vi "Joystick and Camera.vi"() -> ()   [LabVIEW 2016]
uses:
  Classes/Controller/Camera/Machine Vision.ctl
  Classes/Controller/I-O/I-O.lvclass
  Classes/Controller/Motion/Motion.lvclass
  Classes/Controller/Camera/Camera.lvclass
  Classes/Controller/Controller.lvclass
panel:
  out "x .and. y?":bool
  out "Array":dbl[](array[numeric])
  out "array w/ subset deleted":dbl[](array[numeric])
  in  "Go 3":bool
  in  "light":dbl=5.0
  in  "Change light":bool
  out "XYZTheta Out":dbl[](array[numeric])
  in  "Machine Vision":T1
  in  "Move 10cm Right":bool
  in  "Move 10cm Backward":bool
  in  "Move 10cm Forward":bool
  in  "Move 10cm Left":bool
  in  "Record Measurement":bool=TRUE
  in  "Dismount Silicon Tray":bool
  in  "Secure Silicon Tray":bool
  in  "Z Go":bool
  in  "Position":dbl
  in  "XYZTheta":dbl[](array[numeric])
  in  "Go":bool
  in  "Joystick":bool
  out "Sum":dbl[](array[numeric])
  out "Gantry":dbl[](array[numeric])
  in  "Stop":bool
  out "Image":T2(plugin-control)
  out "Camera":dbl[](array[numeric])
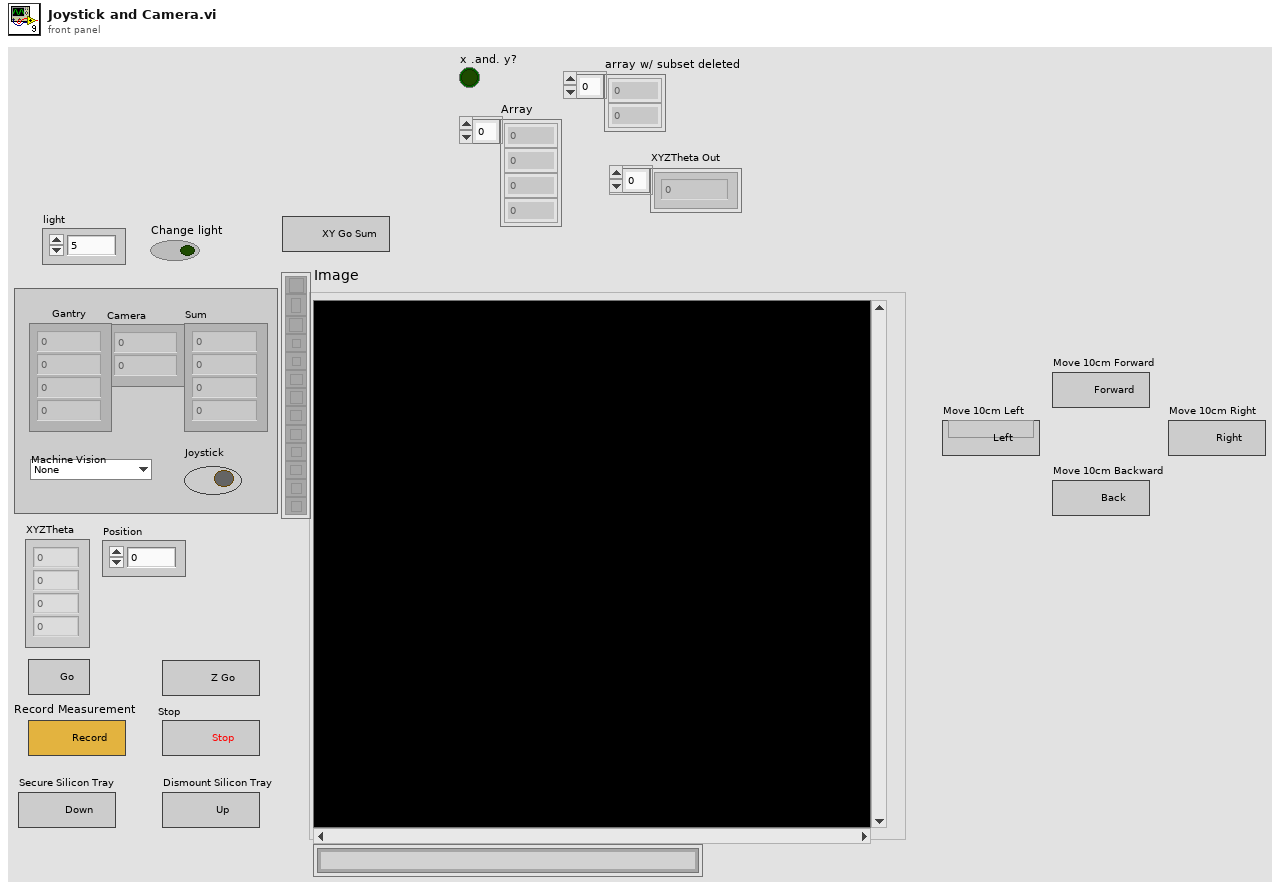
[diagram p1: front panel]
types:
  T1 = typedef "Camera.lvclass/Machine Vision.ctl" = enum16{"None", "Circle", "Tray Fiducials", "Tray Fiducials, top right", "HPK Silicon", "Hexaboard", "Corner (TL, BR)", "Corner (BL, TR)"}
  T2 = typedef "IMAQ Image.ctl" = refnum<image>
  T3 = typedef "Controller.lvclass/Controllers.ctl" = cluster{"I-O.lvclass":refnum<class "I-O.lvclass">, "Motion.lvclass":refnum<class "Motion.lvclass">, "Dispenser.lvclass":refnum<class "Dispenser.lvclass">}
  T4 = typedef "I-O.lvclass/Pin Map.ctl" = cluster{"Region Valves":i32[], "Extra Valves":dbl[][][], "Tool Primary Valve":i32, "Tool Secondary Valve":i32, "Region Sensors":i32[], "Extra Sensors":dbl[][][], "Tool Primary Sensor":dbl, "Tool Secondary Sensor":dbl, "Compression Sensor":dbl, "5V":i32}
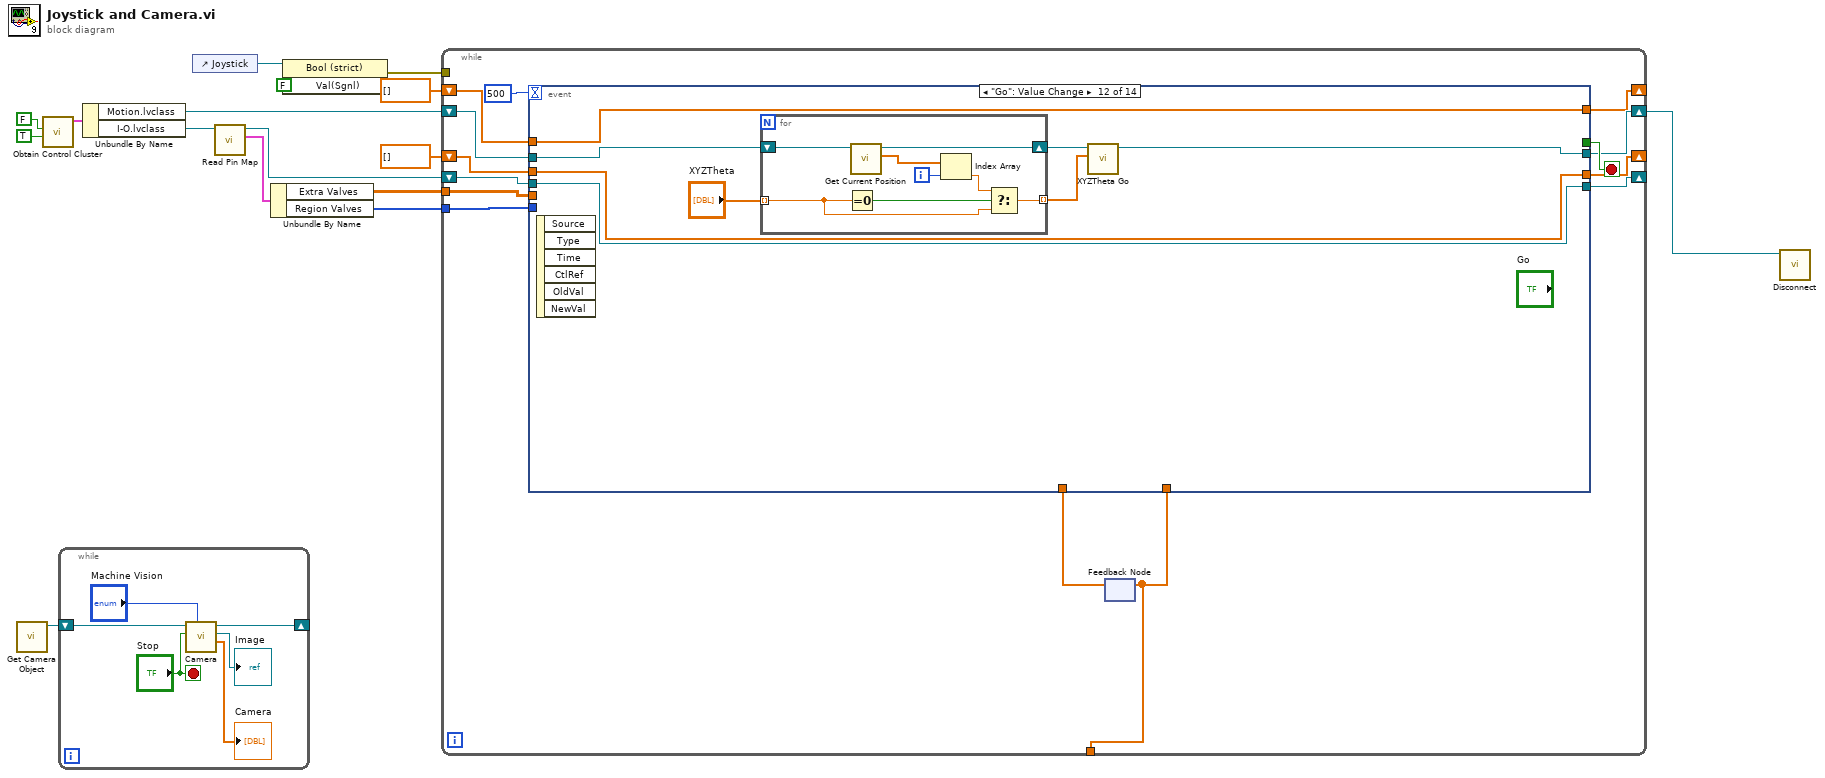
[diagram p0: block diagram]
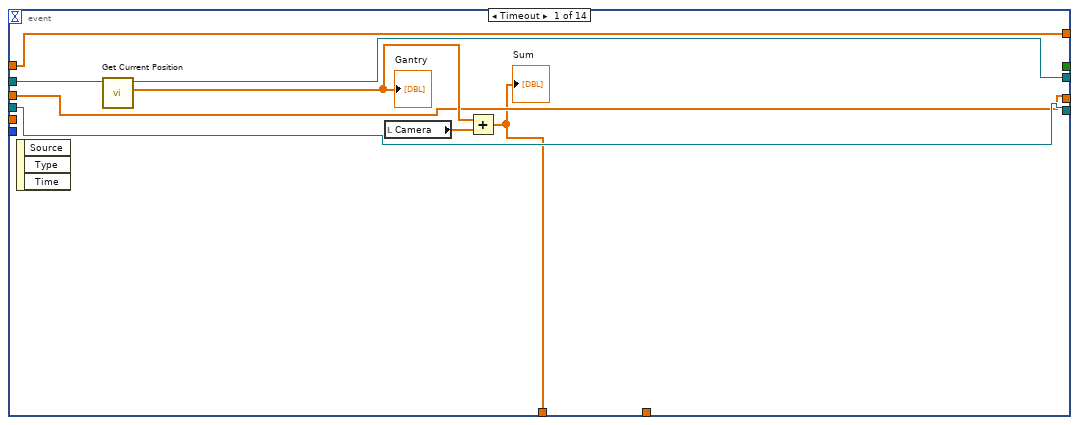
[diagram p2: hidden frame]
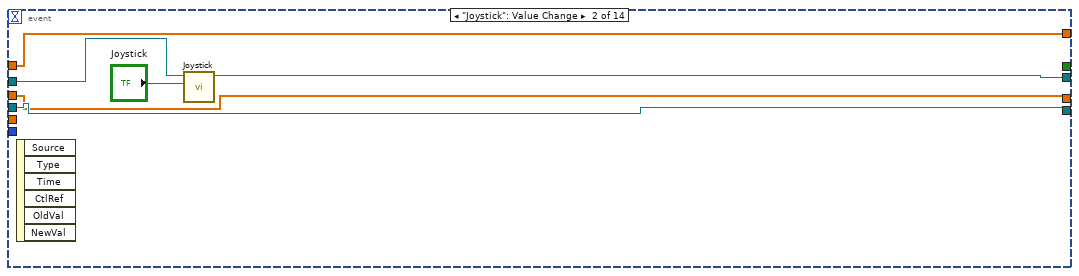
[diagram p3: hidden frame]
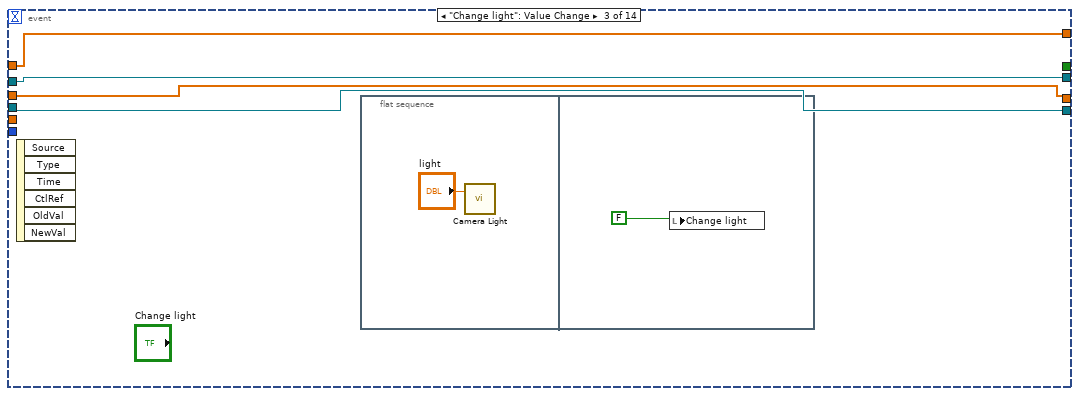
[diagram p4: hidden frame]
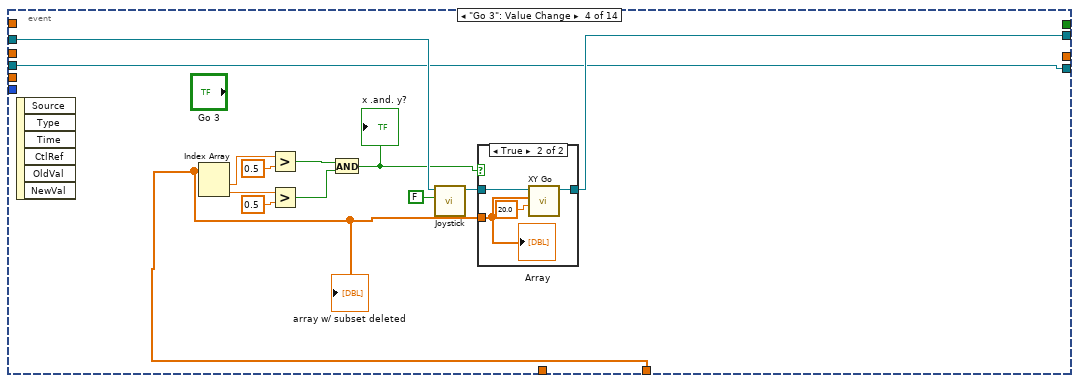
[diagram p5: hidden frame]
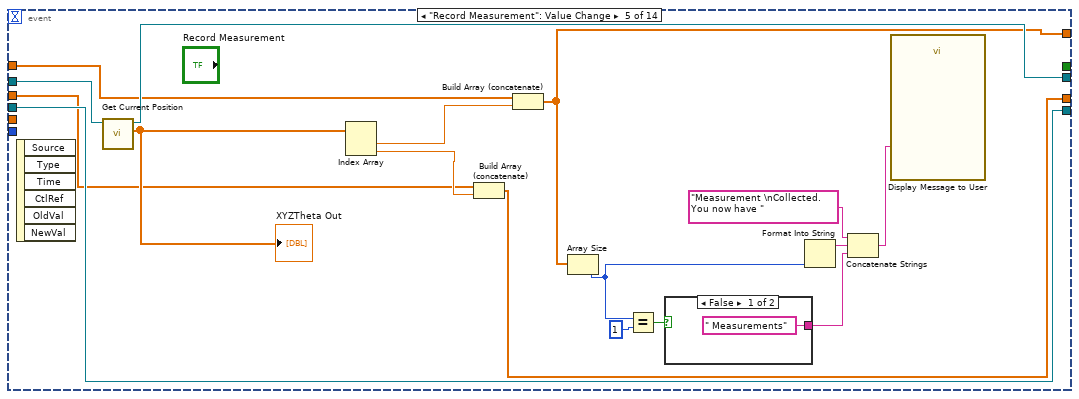
[diagram p7: hidden frame]
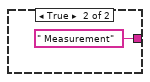
[diagram p8: hidden frame]
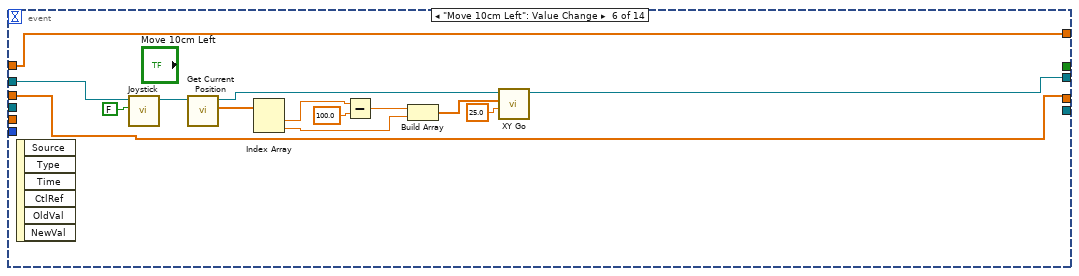
[diagram p9: hidden frame]
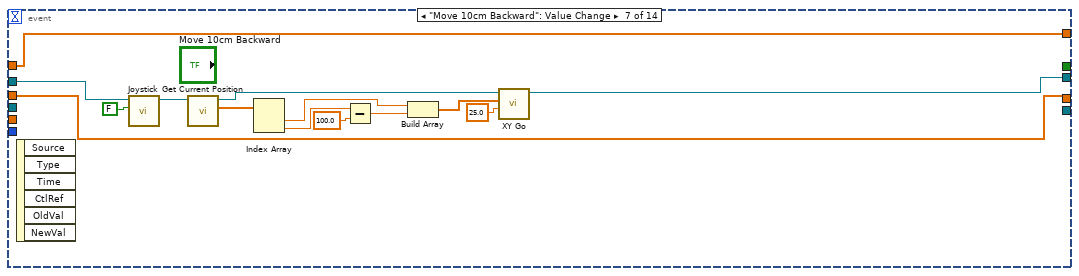
[diagram p10: hidden frame]
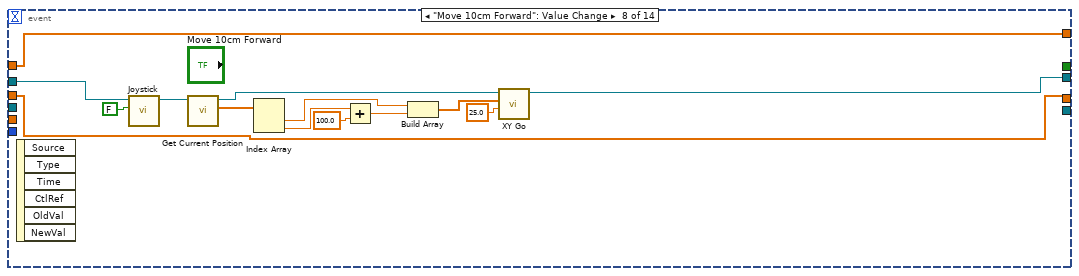
[diagram p11: hidden frame]
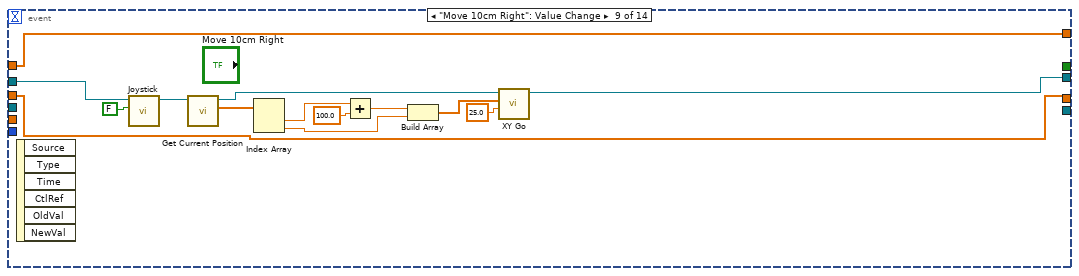
[diagram p12: hidden frame]
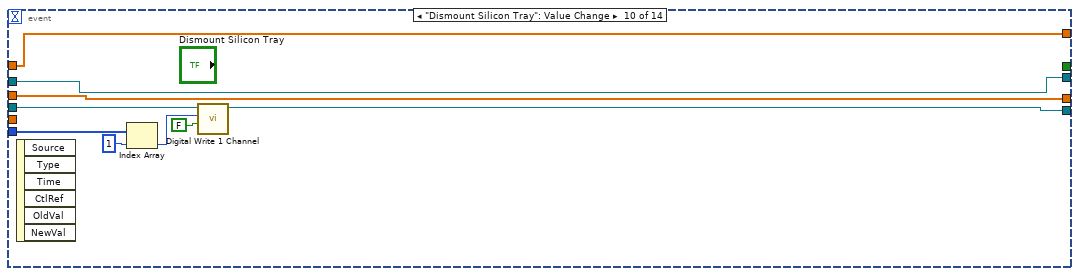
[diagram p13: hidden frame]
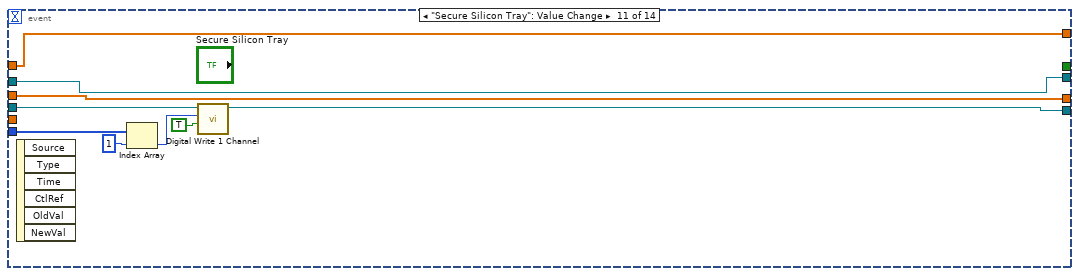
[diagram p14: hidden frame]
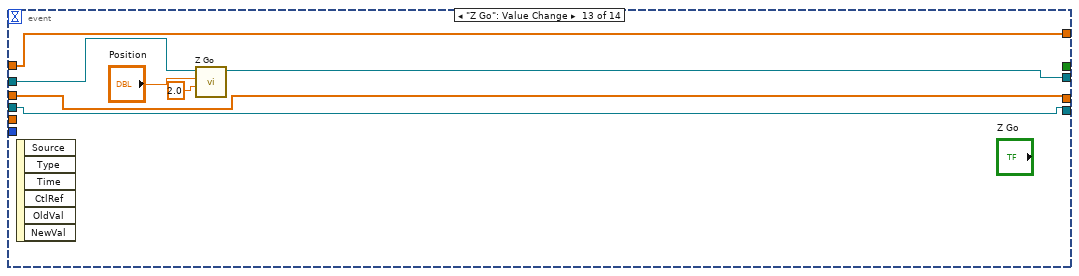
[diagram p15: hidden frame]
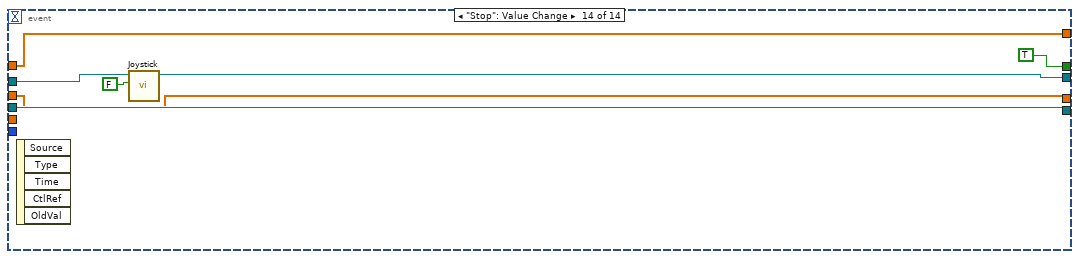
[diagram p16: hidden frame]
diagram:
  n1 = call "Get Camera Object.vi"() -> ("Camera out"=w8:refnum<class "Camera.lvclass">)  [unwired: 10 in, 1 out]
  n2 = call "Obtain Control Cluster.vi"("I/O"=TRUE, "Dispense"=FALSE) -> ("Control Out"=w10:T3)  [unwired: 9 in]
  n3 = while {
    shift-right: [w21] -> _
    shift-left: w8 -> [w22]
    stop <- "Stop" stop-if-true
    n4 = call "Camera.vi"("Machine Vision"="Machine Vision", "Stop"="Stop", "Camera in"=w22) -> ("Camera"=→"Camera":dbl[], "Image"=→"Image":T2, "Camera out"=w21:refnum<class "Camera.lvclass">)  [unwired: 5 in, 1 out]
  }
  n5 = Unbundle By Name(w10) -> ("Motion.lvclass"=w9:refnum<class "Motion.lvclass">, "I-O.lvclass"=w7:refnum<class "I-O.lvclass">)
  n6 = control-ref of="Joystick"() -> (w15:refnum<vi>)
  n7 = call-dynamic "Read Pin Map.vi"("I-O in"=w7) -> ("Pin Map 2"=w5:T4, "I-O out"=w6:refnum<class "I-O.lvclass">)  [unwired: 8 in, 1 out]
  n8 = Unbundle By Name(w5) -> ("Extra Valves"=w3:dbl[][][], "Region Valves"=w4:i32[])
  n9 = property class="Bool (strict)"(reference=w15, "Val(Sgnl)"=FALSE ("Value (Signaling)")) -> (error out=w13:errorcluster)  [unwired: 1 in, 1 out]
  n10 = while {
    shift-right: [w33] -> w14
    shift-left: w9 -> [w34]
    tunnel: w13 -> [_]
    shift-right: [w31] -> _
    shift-left: w6 -> [w32]
    tunnel: w4 -> [w30]
    tunnel: w3 -> [w29]
    shift-right: [w26] -> _
    shift-left: dbl[] [] -> [w28]
    shift-right: [w25] -> _
    shift-left: dbl[] [] -> [w27]
    tunnel: [w23] -> _
    stop <- w35 stop-if-true
    n11 = feedback #1() -> (w23:dbl[])  [unwired: 1 in]
    n12 = event shown="[11] \"Go\": Value Change" {
      selector: _ -> [_ _ _ _ _ _ _ _ _ _ _ _ _ _]
      dyn-events: _ -> [_ _ _ _ _ _ _ _ _ _ _ _ _ _]
      timeout: 500 -> [_ _ _ _ _ _ _ _ _ _ _ _ _ _]
      tunnel: [_ _ _ _ _ _ _ _ _ _ _ _ _ TRUE] -> w35
      tunnel: w34 -> [w43 w50 w54 w69 w91 w98 w111 w125 w139 w152 w166 w174 w190 w196]
      tunnel: [w42 w48 w54 w67 w90 w99 w118 w130 w142 w152 w166 w171 w189 w194] -> w33
      tunnel: w32 -> [w41 w47 w53 w58 w89 _ _ _ _ w156 w167 w170 w186 w193]
      tunnel: [w41 w47 w53 w58 w89 _ _ _ _ w153 w161 w170 w186 w193] -> w31
      tunnel: w30 -> [_ _ _ _ _ _ _ _ _ w158 w165 _ _ _]
      tunnel: w29 -> [_ _ _ _ _ _ _ _ _ _ _ _ _ _]
      tunnel: w28 -> [w39 w46 w51 _ w75 w95 w109 w123 w137 w151 w160 w169 w185 w192]
      tunnel: [w39 w46 w51 _ w79 w95 w109 w123 w137 w151 w160 w169 w185 w192] -> w26
      tunnel: w27 -> [w38 w45 w52 _ w76 w94 w108 w122 w136 w150 w159 w168 w184 w191]
      tunnel: [w38 w45 w52 _ w78 w94 w108 w122 w136 w150 w159 w168 w184 w191] -> w25
      tunnel: [w37 _ _ _ _ _ _ _ _ _ _ _ _ _] -> w24
      tunnel: w23 -> [_ _ _ w57 _ _ _ _ _ _ _ _ _ _]
      event Timeout {
        n13 = event-data() -> ()  [unwired: 1 in, 3 out]
        n14 = call-dynamic "Get Current Position.vi"("Motion in"=w43) -> ("XYZTheta Out"=w40:dbl[], "Motion out"=w42:refnum<class "Motion.lvclass">)  [unwired: 8 in, 1 out]
        "Gantry" <- w40
        n15 = local read "Camera"() -> (w44:dbl[])
        n16 = Add(x=w40, y=w44) -> (x+y=w37:dbl[])
        "Sum" <- w37
      }
      event "Joystick": Value Change {
        n17 = event-data() -> ()  [unwired: 1 in, 6 out]
        n18 = call-dynamic "Joystick.vi"("Joystick"="Joystick", "Motion in"=w50) -> ("Motion out"=w48:refnum<class "Motion.lvclass">)  [unwired: 8 in, 1 out]
      }
      event "Change light": Value Change {
        n19 = event-data() -> ()  [unwired: 1 in, 6 out]
        n20 = flat-sequence {
          frame #0 {
            n21 = call "Camera Light.vi"("input"="light") -> ()  [unwired: 2 in, 1 out]
          }
          frame #1 {
            n22 = local write "Change light"(FALSE) -> ()
          }
        }
      }
      event "Go 3": Value Change {
        n23 = event-data() -> ()  [unwired: 1 in, 6 out]
        n24 = Index Array(array=w57) -> (element #1=w61:dbl, element #2=w60:dbl)  [unwired: 2 in]
        n25 = Greater?(x=w61, y=0.5) -> (0:w64:bool)
        n26 = Greater?(x=w60, y=0.5) -> (0:w63:bool)
        n27 = And(x=w64, y=w63) -> (x .and. y?=w62:bool)
        "x .and. y?" <- w62
        n28 = call-dynamic "Joystick.vi"("Joystick"=FALSE, "Motion in"=w69) -> ("Motion out"=w68:refnum<class "Motion.lvclass">)  [unwired: 8 in, 1 out]
        n29 = case shown="True" w62 {
          tunnel: w68 -> [w70 w74]
          tunnel: [w70 w73] -> w67
          tunnel: w57 -> [_ w72]
          frame False {
          }
          frame True {
            n30 = call-dynamic "XY Go.vi"("Speed"=20.0, "XY"=w72, "Motion in"=w74) -> ("Motion out"=w73:refnum<class "Motion.lvclass">)  [unwired: 7 in, 1 out]
            "Array" <- w72
          }
        }
        "array w/ subset deleted" <- w57
      }
      event "Record Measurement": Value Change {
        n31 = event-data() -> ()  [unwired: 1 in, 6 out]
        n32 = call-dynamic "Get Current Position.vi"("Motion in"=w91) -> ("XYZTheta Out"=w80:dbl[], "Motion out"=w90:refnum<class "Motion.lvclass">)  [unwired: 8 in, 1 out]
        "XYZTheta Out" <- w80
        n33 = Index Array(array=w80) -> (element #1=w88:dbl, element #2=w77:dbl)  [unwired: 2 in]
        n34 = Build Array (concatenate)(w75, w77) -> (w79:dbl[])
        n35 = Build Array (concatenate) "Build Array"(w76, w88) -> (w78:dbl[])
        n36 = Array Size(array=w78) -> (size(s)=w83:i32)
        n37 = Equal?(x=w83, y=1) -> (x = y?=w82:bool)
        n38 = case shown="False" w82 {
          tunnel: [" Measurements" " Measurement"] -> w81
          frame False {
          }
          frame True {
          }
        }
        n39 = Format Into String(w83) -> (resulting string=w87:string)  [unwired: 3 in, 1 out]
        n40 = Concatenate Strings("Measurement \nCollected. You now have ", w87, w81) -> (w85:string)
        n41 = call "Display Message to User"("Message"=w85) -> ()  [unwired: 9 in, 2 out]
      }
      event "Move 10cm Left": Value Change {
        n42 = event-data() -> ()  [unwired: 1 in, 6 out]
        n43 = call-dynamic "Joystick.vi"("Joystick"=FALSE, "Motion in"=w98) -> ("Motion out"=w97:refnum<class "Motion.lvclass">)  [unwired: 8 in, 1 out]
        n44 = call-dynamic "Get Current Position.vi"("Motion in"=w97) -> ("XYZTheta Out"=w106:dbl[], "Motion out"=w107:refnum<class "Motion.lvclass">)  [unwired: 8 in, 1 out]
        n45 = Index Array(array=w106) -> (element #1=w105:dbl, element #2=w102:dbl)  [unwired: 2 in]
        n46 = Subtract(x=w105, y=100.0) -> (x-y=w103:dbl)
        n47 = Build Array(w103, w102) -> (w101:dbl[])
        n48 = call-dynamic "XY Go.vi"("Speed"=25.0, "XY"=w101, "Motion in"=w107) -> ("Motion out"=w99:refnum<class "Motion.lvclass">)  [unwired: 7 in, 1 out]
      }
      event "Move 10cm Backward": Value Change {
        n49 = event-data() -> ()  [unwired: 1 in, 6 out]
        n50 = call-dynamic "Joystick.vi"("Joystick"=FALSE, "Motion in"=w111) -> ("Motion out"=w110:refnum<class "Motion.lvclass">)  [unwired: 8 in, 1 out]
        n51 = call-dynamic "Get Current Position.vi"("Motion in"=w110) -> ("XYZTheta Out"=w120:dbl[], "Motion out"=w121:refnum<class "Motion.lvclass">)  [unwired: 8 in, 1 out]
        n52 = Index Array(array=w120) -> (element #1=w114:dbl, element #2=w117:dbl)  [unwired: 2 in]
        n53 = Subtract(x=w117, y=100.0) -> (x-y=w115:dbl)
        n54 = Build Array(w114, w115) -> (w113:dbl[])
        n55 = call-dynamic "XY Go.vi"("Speed"=25.0, "XY"=w113, "Motion in"=w121) -> ("Motion out"=w118:refnum<class "Motion.lvclass">)  [unwired: 7 in, 1 out]
      }
      event "Move 10cm Forward": Value Change {
        n56 = event-data() -> ()  [unwired: 1 in, 6 out]
        n57 = call-dynamic "Joystick.vi"("Joystick"=FALSE, "Motion in"=w125) -> ("Motion out"=w124:refnum<class "Motion.lvclass">)  [unwired: 8 in, 1 out]
        n58 = call-dynamic "Get Current Position.vi"("Motion in"=w124) -> ("XYZTheta Out"=w134:dbl[], "Motion out"=w135:refnum<class "Motion.lvclass">)  [unwired: 8 in, 1 out]
        n59 = Index Array(array=w134) -> (element #1=w128:dbl, element #2=w129:dbl)  [unwired: 2 in]
        n60 = Add(x=w129, y=100.0) -> (x+y=w127:dbl)
        n61 = Build Array(w128, w127) -> (w132:dbl[])
        n62 = call-dynamic "XY Go.vi"("Speed"=25.0, "XY"=w132, "Motion in"=w135) -> ("Motion out"=w130:refnum<class "Motion.lvclass">)  [unwired: 7 in, 1 out]
      }
      event "Move 10cm Right": Value Change {
        n63 = event-data() -> ()  [unwired: 1 in, 6 out]
        n64 = call-dynamic "Joystick.vi"("Joystick"=FALSE, "Motion in"=w139) -> ("Motion out"=w138:refnum<class "Motion.lvclass">)  [unwired: 8 in, 1 out]
        n65 = call-dynamic "Get Current Position.vi"("Motion in"=w138) -> ("XYZTheta Out"=w148:dbl[], "Motion out"=w149:refnum<class "Motion.lvclass">)  [unwired: 8 in, 1 out]
        n66 = Index Array(array=w148) -> (element #1=w141:dbl, element #2=w145:dbl)  [unwired: 2 in]
        n67 = Add(x=w141, y=100.0) -> (x+y=w146:dbl)
        n68 = Build Array(w146, w145) -> (w144:dbl[])
        n69 = call-dynamic "XY Go.vi"("Speed"=25.0, "XY"=w144, "Motion in"=w149) -> ("Motion out"=w142:refnum<class "Motion.lvclass">)  [unwired: 7 in, 1 out]
      }
      event "Dismount Silicon Tray": Value Change {
        n70 = event-data() -> ()  [unwired: 1 in, 6 out]
        n71 = Index Array(array=w158, index=1) -> (element=w155:i32)
        n72 = call-dynamic "Digital Write 1 Channel.vi"("Value"=FALSE, "Channel"=w155, "I-O.lvclass"=w156) -> ("I-O.lvclass 2"=w153:refnum<class "I-O.lvclass">)  [unwired: 7 in, 1 out]
      }
      event "Secure Silicon Tray": Value Change {
        n73 = event-data() -> ()  [unwired: 1 in, 6 out]
        n74 = Index Array(array=w165, index=1) -> (element=w163:i32)
        n75 = call-dynamic "Digital Write 1 Channel.vi"("Value"=TRUE, "Channel"=w163, "I-O.lvclass"=w167) -> ("I-O.lvclass 2"=w161:refnum<class "I-O.lvclass">)  [unwired: 7 in, 1 out]
      }
      event "Go": Value Change {
        n76 = event-data() -> ()  [unwired: 1 in, 6 out]
        n77 = for {
          tunnel: "XYZTheta" -> [w181] mode=indexing
          tunnel: [w179] -> w173 mode=indexing
          shift-right: [w177] -> w172
          shift-left: w174 -> [w178]
          i -> [w183]
          n78 = Equal To 0?(x=w181) -> (x = 0?=w182:bool)
          n79 = call-dynamic "Get Current Position.vi"("Motion in"=w178) -> ("XYZTheta Out"=w176:dbl[], "Motion out"=w177:refnum<class "Motion.lvclass">)  [unwired: 8 in, 1 out]
          n80 = Index Array(array=w176, index=w183) -> (element=w180:dbl)
          n81 = Select(t=w180, s=w182, f=w181) -> (s? t:f=w179:dbl)
        }
        n82 = call "XYZTheta Go.vi"("XYZTheta In"=w173, "Motion in"=w172) -> ("Motion out"=w171:refnum<class "Motion.lvclass">)  [unwired: 7 in, 2 out]
      }
      event "Z Go": Value Change {
        n83 = event-data() -> ()  [unwired: 1 in, 6 out]
        n84 = call-dynamic "Z Go.vi"("Speed"=2.0, "Position"="Position", "Motion in"=w190) -> ("Motion out"=w189:refnum<class "Motion.lvclass">)  [unwired: 7 in, 1 out]
      }
      event "Stop": Value Change {
        n85 = event-data() -> ()  [unwired: 1 in, 5 out]
        n86 = call-dynamic "Joystick.vi"("Joystick"=FALSE, "Motion in"=w196) -> ("Motion out"=w194:refnum<class "Motion.lvclass">)  [unwired: 8 in, 1 out]
      }
    }
    n87 = feedback-in #1(w24) -> ()
  }
  n88 = call-dynamic "Disconnect.vi"("Controller in"=w14) -> ()  [unwired: 9 in, 1 out]
